vi "WriteBase.vi"(0 "National Instruments USB-8473 Adapter Class in":refnum<class "National Instruments USB-8473 Adapter Class.lvclass">, 5 "Id":u32 format="%08x", 7 "DataLength":i32, 9 "Data":u8[](array[numeric]) format="%02x", 11 "error in (no error)":errorcluster) -> (4 "National Instruments USB-8473 Adapter Class out":refnum<class "National Instruments USB-8473 Adapter Class.lvclass">, 15 "error out":errorcluster)   [LabVIEW 2011, in "National Instruments USB-8473 Adapter Class.lvclass"]
uses:
  National Instruments USB-8473 Adapter Class.lvclass
  National Instruments USB-8473 Adapter Class.lvclass/National Instruments USB-8473 Adapter Class.ctl
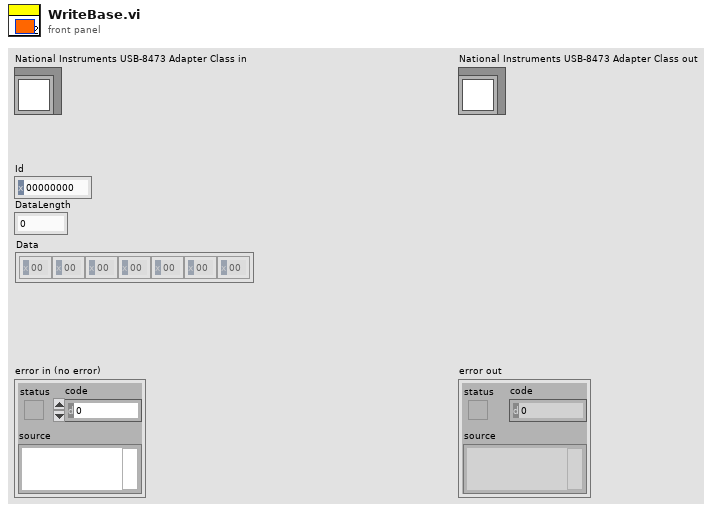
[diagram p1: front panel]
types:
  T1 = typedef "xobjhandle.ctl" = u32
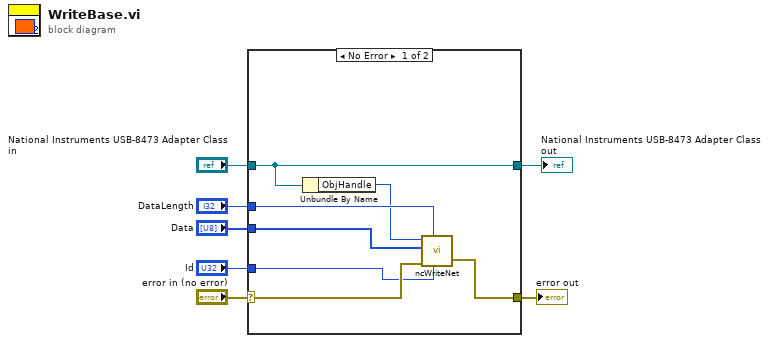
[diagram p0: block diagram]
diagram:
  n1 = case shown="No Error" "error in (no error)" {
    selector: "error in (no error)" -> [w14 w16]
    tunnel: [w9 w16] -> w6
    tunnel: [w8 w15] -> w4
    tunnel: "National Instruments USB-8473 Adapter Class in" -> [w8 w15]
    tunnel: "Id" -> [w13 _]
    tunnel: "DataLength" -> [w12 _]
    tunnel: "Data" -> [w11 _]
    frame No Error {
      n2 = Unbundle By Name(w8) -> ("ObjHandle"=w10:T1)
      n3 = call <vilib>:"ncWriteNet.vi"("ArbitrationId"=w13, "DataLength"=w12, "Error in"=w14, "Data"=w11, "ObjHandle in"=w10) -> ("Error out"=w9:errorcluster)  [unwired: 1 in, 1 out]
    }
    frame Error {
    }
  }
  "error out" <- w6
  "National Instruments USB-8473 Adapter Class out" <- w4
